vi "Test Create.vi"(11 "Test Case In":refnum<class "Test Open Xml.lvclass">) -> (0 "error out":errorcluster, 3 "Test Case Out":refnum<class "Test Open Xml.lvclass">)   [LabVIEW 2020, in "Test Open Xml.lvclass"]
uses:
  Test Open Xml.lvclass
  Source/Open Xml.lvlib
  <vilib>/Astemes/LUnit/Test Case.lvclass
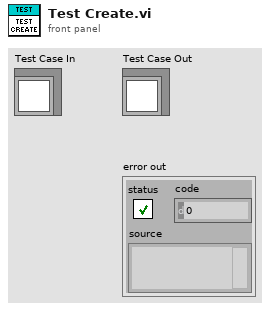
[diagram p1: front panel]
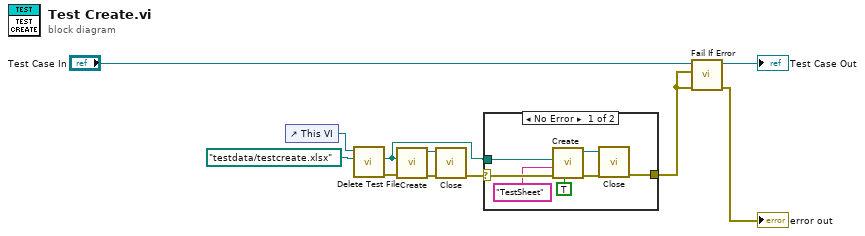
[diagram p0: block diagram]
diagram:
  n1 = control-ref of="This VI"() -> (w3:refnum<vi>)
  n2 = call "Delete Test File.vi"("name or relative path"=path "testdata/testcreate.xlsx", "VI in"=w3) -> ("error out"=w4:errorcluster, "deleted path"=w1:path)  [unwired: 8 in]
  n3 = call "Create.vi"("error in"=w4, "Path"=w1) -> ("error out"=w8:errorcluster, "SpreadsheetDoc"=w7:refnum<k24>)  [unwired: 8 in]
  n4 = call "Close.vi"("error in"=w8, "SpreadsheetDoc"=w7) -> ("error out"=w6:errorcluster)  [unwired: 9 in]
  n5 = case shown="No Error" w6 {
    selector: w6 -> [w18 w19]
    tunnel: w1 -> [w15 _]
    tunnel: [w13 w19] -> w5
    frame No Error {
      n6 = call "Create.vi"("Overwrite?"=TRUE, "error in"=w18, "SheetName"="TestSheet", "Path"=w15) -> ("error out"=w17:errorcluster, "SpreadsheetDoc"=w16:refnum<k24>)  [unwired: 6 in]
      n7 = call "Close.vi"("error in"=w17, "SpreadsheetDoc"=w16) -> ("error out"=w13:errorcluster)  [unwired: 9 in]
    }
    frame Error {
    }
  }
  n8 = call <vilib>:"Fail If Error.vi"("error in (no error)"=w5, "Assert error"=w5, "LUnit Test Case In"="Test Case In") -> ("error out"=→"error out":errorcluster, "LUnit Test Case Out"=→"Test Case Out":refnum<class "Test Open Xml.lvclass">)  [unwired: 7 in]
